vi "Configure Transition Time.vi"(0 "VISA resource name":refnum<visa-resource-name>, 1 "Delay (0.5 s)":dbl=0.5 min=0.5 max=999.9 format="%.1f", 5 "Ramp Up Time (0 s)":dbl min=0.0 max=999.9 format="%.1f", 7 "Dwell (1 s)":dbl=1.0 min=0.5 max=999.9 format="%.1f", 9 "Ramp Down Time (0 s)":dbl min=0.0 max=999.9 format="%.1f", 11 "error in (no error)":errorcluster) -> (4 "VISA resource name out":refnum<visa-resource-name>, 15 "error out":errorcluster)   [LabVIEW 2014, in "eec 6700.lvlib"]
doc: "Configures the ramp up time, dwell time, delay time, ramp down time</B> in the active memory of the power source instrument.\n\nNote : This VI should be used in the Program mode only.\nRun \"Configure Program Mode.vi\" to make sure the instrument is in <B>Program Mode</B> before using this VI"
uses:
  <instrlib>/eec 6700/eec 6700.lvlib
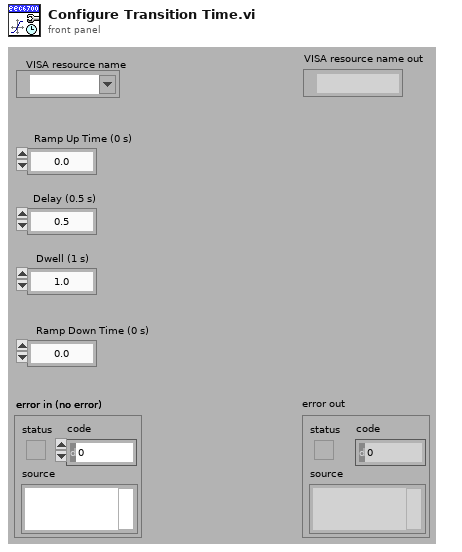
[diagram p1: front panel]
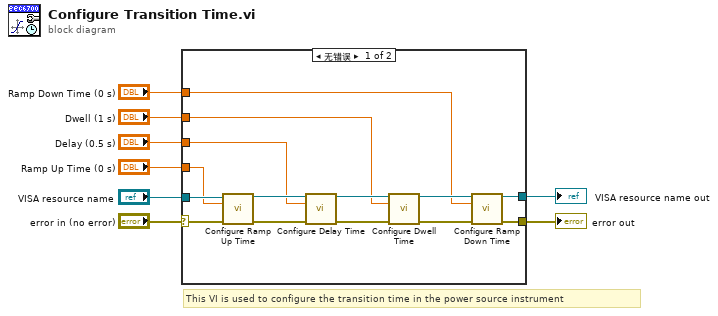
[diagram p0: block diagram]
diagram:
  # "This VI is used to configure the transition time in the power source instrument"
  n1 = case shown="无错误" "error in (no error)" {
    selector: "error in (no error)" -> [w13 w24]
    tunnel: [w22 w24] -> w8
    tunnel: [w21 w23] -> w7
    tunnel: "VISA resource name" -> [w14 w23]
    tunnel: "Ramp Down Time (0 s)" -> [w12 _]
    tunnel: "Dwell (1 s)" -> [w11 _]
    tunnel: "Delay (0.5 s)" -> [w10 _]
    tunnel: "Ramp Up Time (0 s)" -> [w9 _]
    frame No Error {
      n2 = call <instrlib>:"Configure Ramp Up Time.vi"("VISA resource name"=w14, "Ramp Up Time (0 s)"=w9, "error in (no error)"=w13) -> ("VISA resource name out"=w15:refnum<visa-resource-name>, "error out"=w20:errorcluster)  [unwired: 11 in]
      n3 = call <instrlib>:"Configure Delay Time.vi"("VISA resource name"=w15, "Delay (0.5 s)"=w10, "error in (no error)"=w20) -> ("VISA resource name out"=w16:refnum<visa-resource-name>, "error out"=w19:errorcluster)  [unwired: 11 in]
      n4 = call <instrlib>:"Configure Dwell Time.vi"("VISA resource name"=w16, "Dwell (1 s)"=w11, "error in (no error)"=w19) -> ("VISA resource name out"=w17:refnum<visa-resource-name>, "error out"=w18:errorcluster)  [unwired: 11 in]
      n5 = call <instrlib>:"Configure Ramp Down Time.vi"("VISA resource name"=w17, "Ramp Down Time (0 s)"=w12, "error in (no error)"=w18) -> ("VISA resource name out"=w21:refnum<visa-resource-name>, "error out"=w22:errorcluster)  [unwired: 11 in]
    }
    frame Error {
    }
  }
  "error out" <- w8
  "VISA resource name out" <- w7
